vi "set_config_cluster.vi"(8 "error in (no error)":errorcluster, 10 "config cluster variant":variant, 11 "StageFH090410SharedVariable in":refnum<class "StageFH090410SharedVariable.lvclass">) -> (0 "error out":errorcluster, 3 "StageFH090410SharedVariable out":refnum<class "StageFH090410SharedVariable.lvclass">)   [LabVIEW 2010, in "StageFH090410SharedVariable.lvclass"]
uses:
  StageFH090410SharedVariable.lvclass
  StageFH090410SharedVariable.lvclass/StageFH090410SharedVariable.ctl
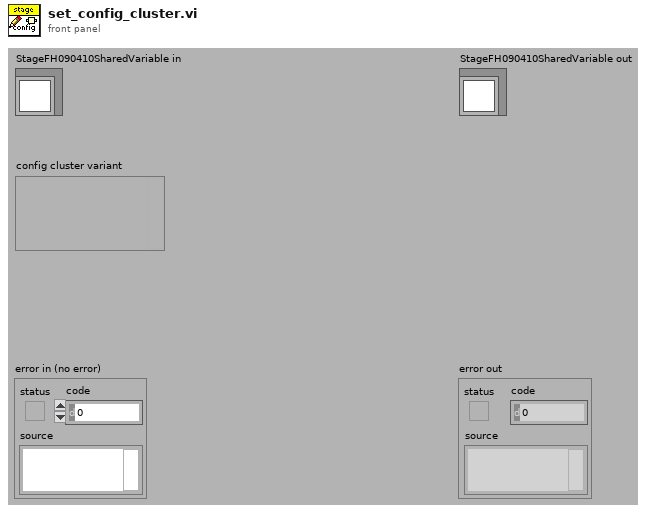
[diagram p1: front panel]
types:
  T1 = typedef "StageFH090410SharedVariable.lvclass/config_data_cluster.ctl" = cluster{"SV command":string, "SV position feedback":string, "SV move trigger":string, "command mode":T2, "tolerance":dbl[unit]}
  T2 = typedef "StageFH090410SharedVariable.lvclass/command_mode_enum.ctl" = enum16{"step", "absolute"}
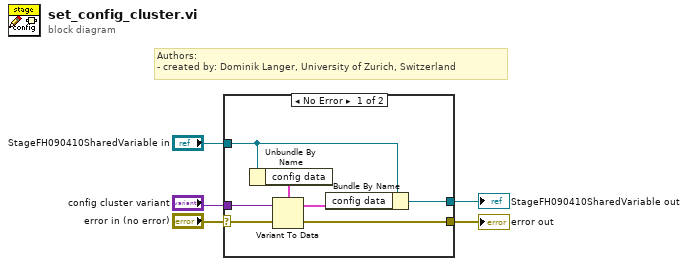
[diagram p0: block diagram]
diagram:
  # "Authors: \n- created by: Dominik Langer, University of Zurich, Switzerland"
  n1 = case shown="No Error" "error in (no error)" {
    selector: "error in (no error)" -> [w12 w13]
    tunnel: "StageFH090410SharedVariable in" -> [w7 w14]
    tunnel: "config cluster variant" -> [w11 _]
    tunnel: [w9 w13] -> w2
    tunnel: [w6 w14] -> w1
    frame No Error {
      n2 = Unbundle By Name(w7) -> ("config data"=w10:T1)
      n3 = Variant To Data(error in=w12, Variant=w11, type=w10) -> (error out=w9:errorcluster, data=w8:T1)
      n4 = Bundle By Name(cluster=w7, "config data"=w8) -> (w6:refnum<class "StageFH090410SharedVariable.lvclass">)
    }
    frame Error {
    }
  }
  "error out" <- w2
  "StageFH090410SharedVariable out" <- w1
